vi "Version 1_Read Tare Settings.vi"(7 "Address (A)":string="A", 8 "error in":errorcluster, 11 "VISA Session In":refnum<visa-resource-name>="Alicat") -> (0 "error out":errorcluster, 1 "ValveDrive Report":enum32{"Disable", "Enable", "No Change"}(radio)=enum."No Change", 2 "Tare Functions":T1={"Display"=enum."None", "External"=enum."None", "Auto Delay"=nan} {"Auto Delay" format="%.1g"}, 3 "VISA Session Out":refnum<visa-resource-name>, 4 "Totalizer Timer":enum32{"Disable", "Enable", "No Change"}(radio)=enum."No Change")   [LabVIEW 2016]
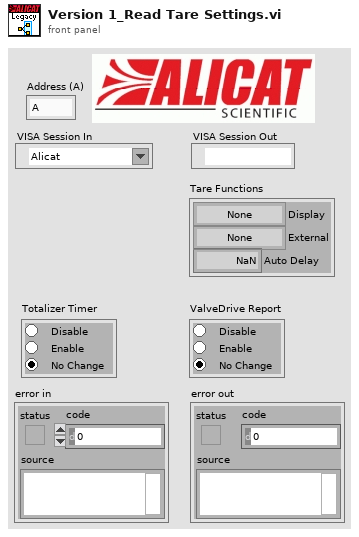
[diagram p1: front panel]
types:
  T1 = cluster{"Display":enum16{"None", "Pressure", "Volumetric"}, "External":enum16{"None", "Pressure", "Volumetric", "Totalizer"}, "Auto Delay":dbl}
  T2 = cluster{"Display":enum16{"None", "Pressure", "Volumetric"}, "External":enum16{"None", "Pressure", "Volumetric", "Totalizer"}, "Auto-Tare Delay [s]":dbl}
  T3 = typedef "Data Frame.ctl" = cluster{"Absolute Pressure":bool, "Gauge/Diff. Pressure":bool, "Barometric Pressure":bool, "Temperature":bool, "Volumetric":bool, "Mass":bool, "Setpoint":bool, "Valve Drive":bool, "Totalizer":bool, "Totalizer Timer":bool, "Totalizer Average Flow":bool, "Totalizer Peak Flow":bool, "Gas Selected":bool, "Tot. Timer Format":u16}
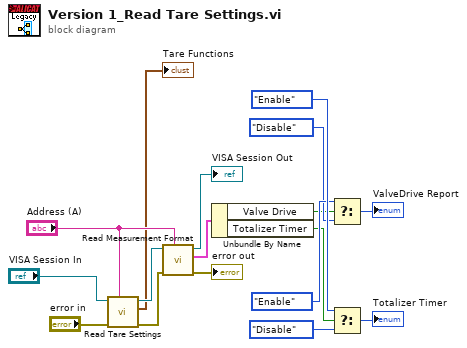
[diagram p0: block diagram]
diagram:
  n1 = call "Read Tare Settings.vi"("Unit ID (A)"="Address (A)", "error in"="error in", "VISA Session In"="VISA Session In") -> ("error out"=w15:errorcluster, "Tare Functions"=→"Tare Functions":T2, "VISA Session Out"=w13:refnum<visa-resource-name>)  [unwired: 6 in]
  n2 = call "Read Measurement Format.vi"("Unit ID (A)"="Address (A)", "error in"=w15, "VISA Session In"=w13) -> ("error out"=→"error out":errorcluster, "Data Frame Format"=w10:T3, "VISA Session Out"=→"VISA Session Out":refnum<visa-resource-name>)  [unwired: 6 in]
  n3 = Unbundle By Name(w10) -> ("Valve Drive"=w3:bool, "Totalizer Timer"=w2:bool)
  n4 = Select(t=enum32{"Disable", "Enable", "No Change"}."Enable" ("ValveDrive Report"), s=w3, f=enum32{"Disable", "Enable", "No Change"}."Disable" ("ValveDrive Report")) -> (s? t:f=→"ValveDrive Report":enum32{"Disable", "Enable", "No Change"})
  n5 = Select(t=enum32{"Disable", "Enable", "No Change"}."Enable" ("Totalizer Timer"), s=w2, f=enum32{"Disable", "Enable", "No Change"}."Disable" ("Totalizer Timer")) -> (s? t:f=→"Totalizer Timer":enum32{"Disable", "Enable", "No Change"})
